vi "ApplyFinalState.vi"(8 "error in (no error)":errorcluster, 10 "Line Final State":enum16{"Default", "High", "Low", "Same"}[](array[ring]), 11 "Output Bits":u32) -> (0 "error out":errorcluster, 3 "Final Output Bits":u32)   [LabVIEW 2013, in "Pulseblaster.lvclass"]
uses:
  Pulseblaster.lvclass
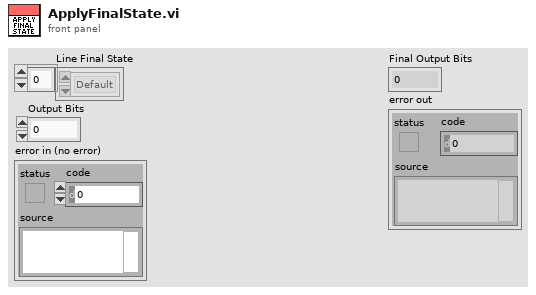
[diagram p1: front panel]
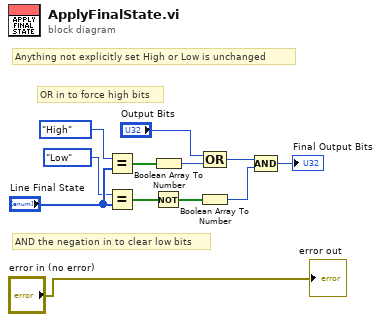
[diagram p0: block diagram]
diagram:
  # "Anything not explicitly set High or Low is unchanged"
  # "OR in to force high bits"
  # "AND the negation in to clear low bits"
  n1 = Equal?(x=enum16{"Default", "High", "Low", "Same"}."High" ("element"), y="Line Final State") -> (x = y?=w8:bool[])
  n2 = Equal?(x=enum16{"Default", "High", "Low", "Same"}."Low" ("element"), y="Line Final State") -> (x = y?=w5:bool[])
  n3 = Not(x=w5) -> (.not. x?=w4:bool[])
  n4 = Boolean Array To Number(Boolean array=w8) -> (number=w7:u32)
  n5 = Boolean Array To Number(Boolean array=w4) -> (number=w3:u32)
  n6 = Compound Arithmetic op=OR("Output Bits", w7) -> (w6:u32)
  n7 = Compound Arithmetic op=AND(w6, w3) -> (→"Final Output Bits":u32)
  "error out" <- "error in (no error)"
